vi "Config IO.vi"(0 "Pulse time us":u32=3 min=3 step=1, 1 "Soft limit enable":bool, 2 "Hard limit enable":bool, 5 "Step idle delay ms (255 keep)":u8=255, 7 "Step pulse invert":T2, 9 "Axis direction":T2, 11 "error in (no error)":errorcluster, 12 "Pins direction":T1) -> (15 "error out":errorcluster)   [LabVIEW 2024, in "GRBL 1.1.lvlib"]
doc: "Step pulse time: Sets time length per step. Minimum 3usec.\nStep idle delay: Sets a short hold delay when stopping to let dynamics settle before disabling steppers. Value 255 keeps motors enabled with no delay.\nStep pulse invert: Inverts the step signal. Set axis bit to invert (00000ZYX).\nStep direction invert: Inverts the direction signal. Set axis bit to invert (00000ZYX).\nInvert step enable pin: Inverts the stepper driver enable pin signal.\nInvert limit pins: Inverts the all of the limit input pins.\nInvert probe pin: Inverts the probe input pin signal.\nSoft limits enable: Enables soft limits checks within machine travel and sets alarm when exceeded. Requires homing.\nHard limits enable: Enables hard limits. Immediately halts motion and throws an alarm when switch is triggered."
uses:
  GRBL 1.1.lvlib
panel:
  out "Data read":string
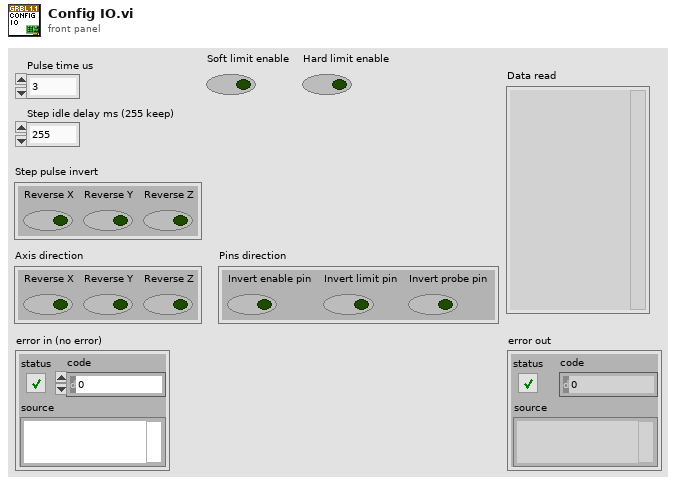
[diagram p1: front panel]
types:
  T1 = cluster{"Invert enable pin":bool, "Invert limit pin":bool, "Invert probe pin":bool}
  T2 = cluster{"Reverse X":bool, "Reverse Y":bool, "Reverse Z":bool}
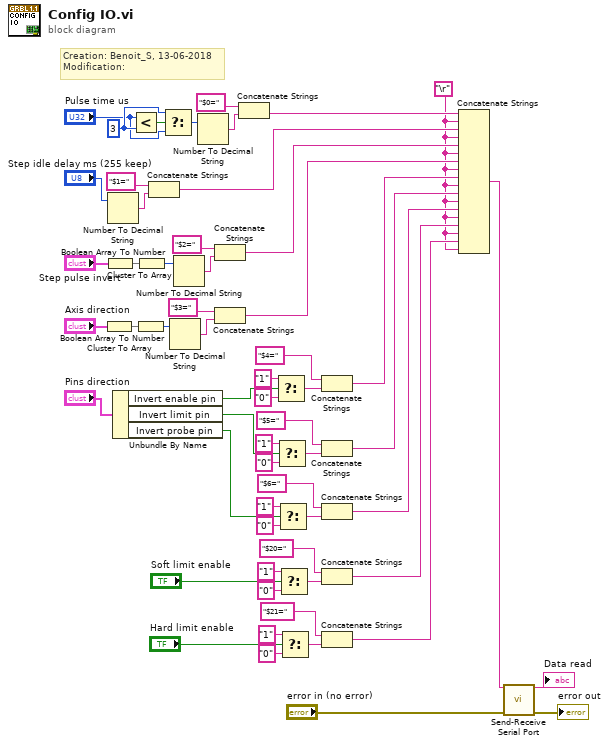
[diagram p0: block diagram]
diagram:
  w3 = "\r"
  w48 = u32 3 ("y")
  # "Creation: Benoit_S, 13-06-2018\nModification:"
  n1 = Cluster To Array(cluster="Axis direction") -> (array=w52:bool[])
  n2 = Cluster To Array(cluster="Step pulse invert") -> (array=w51:bool[])
  n3 = Number To Decimal String(number="Step idle delay ms (255 keep)") -> (decimal integer string=w43:string)  [unwired: 1 in]
  n4 = Unbundle By Name("Pins direction") -> ("Invert enable pin"=w25:bool, "Invert limit pin"=w24:bool, "Invert probe pin"=w23:bool)
  n5 = Less?(x="Pulse time us", y=w48) -> (x < y?=w49:bool)
  n6 = Boolean Array To Number(Boolean array=w52) -> (number=w35:u32)
  n7 = Boolean Array To Number(Boolean array=w51) -> (number=w38:u32)
  n8 = Concatenate Strings("$1=", w43) -> (w11:string)
  n9 = Select(t=w48, s=w49, f="Pulse time us") -> (s? t:f=w46:u32)
  n10 = Number To Decimal String(number=w35) -> (decimal integer string=w37:string)  [unwired: 1 in]
  n11 = Number To Decimal String(number=w38) -> (decimal integer string=w39:string)  [unwired: 1 in]
  n12 = Number To Decimal String(number=w46) -> (decimal integer string=w44:string)  [unwired: 1 in]
  n13 = Concatenate Strings("$2=", w39) -> (w10:string)
  n14 = Concatenate Strings("$3=", w37) -> (w9:string)
  n15 = Concatenate Strings("$0=", w44) -> (w12:string)
  n16 = Select(t="1", s=w25, f="0") -> (s? t:f=w57:string)
  n17 = Select(t="1", s=w24, f="0") -> (s? t:f=w32:string)
  n18 = Select(t="1", s=w23, f="0") -> (s? t:f=w27:string)
  n19 = Select(t="1", s="Soft limit enable", f="0") -> (s? t:f=w21:string)
  n20 = Select(t="1", s="Hard limit enable", f="0") -> (s? t:f=w16:string)
  n21 = Concatenate Strings("$4=", w57) -> (w8:string)
  n22 = Concatenate Strings("$5=", w32) -> (w7:string)
  n23 = Concatenate Strings("$6=", w27) -> (w6:string)
  n24 = Concatenate Strings("$20=", w21) -> (w5:string)
  n25 = Concatenate Strings("$21=", w16) -> (w4:string)
  n26 = Concatenate Strings(w12, w3, w11, w3, w10, w3, w9, w3, w8, w3, w7, w3, w6, w3, w5, w3, w4, w3) -> (w2:string)
  n27 = call "Send-Receive Serial Port.vi"("Data to write"=w2, "error in (no error)"="error in (no error)") -> ("Data read"=→"Data read":string, "error out"=→"error out":errorcluster)  [unwired: 12 in]
